vi "EOL All-Station Module Test Data Buffer.vi"() -> (1 "Store Data out":T1 {"Sun Shade Open Force Limits"."Variance" format="%.2g"; "Sun Shade Open Force Limits"."Truncation End" format="%.2g"; "Sun Shade Open Force Limits"."Truncation Start" format="%.2g"; "Sun Shade Open Force Limits"."Avg Max" format="%.2g"; "Sun Shade Open Force Limits"."Avg Min" format="%.2g"; "Sun Shade Open Force Limits"."Overall Max" format="%.2g"; "Sun Shade Open Force Limits"."Overall Min" format="%.2g"; "Sun Shade Close Force Limits"."Variance" format="%.2g"; "Sun Shade Close Force Limits"."Truncation End" format="%.2g"; "Sun Shade Close Force Limits"."Truncation Start" format="%.2g"; "Sun Shade Close Force Limits"."Avg Max" format="%.2g"; "Sun Shade Close Force Limits"."Avg Min" format="%.2g"; "Sun Shade Close Force Limits"."Overall Max" format="%.2g"; "Sun Shade Close Force Limits"."Overall Min" format="%.2g"; "Motion Data Array"."Motion Data Limits"."LIN Msg"."Msg" format="%02x"; "Motion Data Array"."Motion Data Limits"."LIN Msg"."ID" format="%02x"})   [LabVIEW 2018]
uses:
  02.Type Def's/EOL Save Module Test Data Control.ctl
  02.Type Def's/EOL Motion Database Table.ctl
  02.Type Def's/All Motions.ctl
  05.UserVI's/type defs/17x Audit Motion Data Seq Control.ctl
  05.UserVI's/type defs/17x AP Data Type.ctl
  05.UserVI's/type defs/17x Sunshade Limts Seq.ctl
  02.Type Def's/EOL Module Info Control.ctl
panel:
  # "Min"
  # "N"
  # "Min"
  # "Start"
  # "N"
  # "Max"
  # "N"
  # "Max"
  # "N"
  # "End"
  # "Min"
  # "N"
  # "Min"
  # "Start"
  # "N"
  # "Max"
  # "N"
  # "Max"
  # "N"
  # "End"
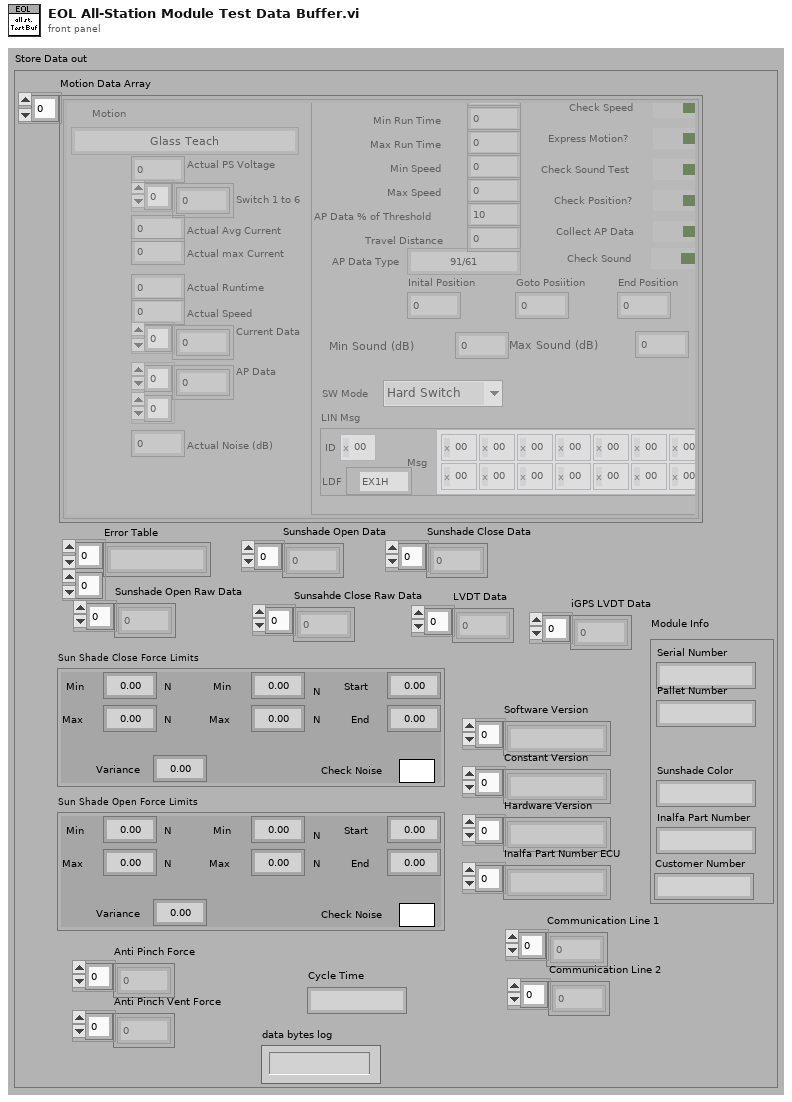
[diagram p1: front panel]
types:
  T1 = typedef "EOL Save Module Test Data Control.ctl" = cluster{"Motion Data Array":T2[], "Error Table":string[][], "Sun Shade Close Force Limits":T6, "Sun Shade Open Force Limits":T6, "Sunshade Open Data":sgl[], "Sunshade Close Data":sgl[], "Module Info":T7, "Sunsahde Close Raw Data":sgl[], "Sunshade Open Raw Data":sgl[], "Software Version":string[], "Constant Version":string[], "Hardware Version":string[], "Inalfa Part Number ECU":string[], "LVDT Data":sgl[], "Communication Line 1":sgl[], "Communication Line 2":sgl[], "Anti Pinch Force":sgl[], "Cycle Time":string, "Anti Pinch Vent Force":sgl[], "iGPS LVDT Data":sgl[], "data bytes log":string}
  T2 = typedef "EOL Motion Database Table.ctl" = cluster{"Motion":T3, "Actual Avg Current":dbl, "Actual Runtime":dbl, "Actual Speed":dbl, "Current Data":sgl[], "Motion Data Limits":T4, "Switch 1 to 6":dbl[], "Actual PS Voltage":dbl, "AP Data":i16[][], "Actual max Current":dbl, "Actual Noise (dB)":dbl}
  T3 = typedef "All Motions.ctl" = enum16{"Glass Teach", "Glass Slide Open", "Glass Slide Close", "Glass Vent Open", "Glass Vent Close", "Sunshade Teach", "Sunshade Open", "Sunshade Close", "Idle", "Sunshade Open 2", "Sunshade Close 2", "Glass Slide Open Sunshade Open", "Glass Slide Open Sunshade Close", "Glass Slide Close Sunshade Open", "Glass Slide Close Sunshade Close", "Glass Vent Open Sunshade Open", "Glass Vent Open Sunshade Close", "Glass Vent Close Sunshade Open", "Glass Vent Close Sunshade Close", "Express Glass Slide Open", "Express Glass Slide Close", "Express Glass Vent Open", "Express Glass Vent Close", "Express Sunshade Open", "Express Sunshade Close", "Express Sunshade Open 2", "Express Sunshade Close 2", "Express Glass Slide Open Sunshade Open", "Express Glass Slide Open Sunshade Close", "Express Glass Slide Close Sunshade Open", "Express Glass Slide Close Sunshade Close", "Express Glass Vent Open Sunshade Open", "Express Glass Vent Open Sunshade Close", "Express Glass Vent Close Sunshade Open", "Express Glass Vent Close Sunshade Close", "Goto Position Glass", "Goto Position Sunshade", "Sunshade Teach 2"}
  T4 = typedef "17x Audit Motion Data Seq Control.ctl" = cluster{"Power Supply Voltage":dbl, "Min Avg Current":dbl, "Max Avg Current":dbl, "Min Run Time":dbl, "Max Run Time":dbl, "Min Speed":dbl, "Max Speed":dbl, "AP Data % of Threshold":dbl, "Travel Distance":dbl, "AP Data Type":T5, "Check Current":bool, "Check Run Time":bool, "Check Speed":bool, "Express Motion?":bool, "Check Sound Test":bool, "Check Position?":bool, "Collect AP Data":bool, "Inital Position":u16, "End Position":u16, "Goto Posiition":u16, "Max max Current":dbl, "Min max Current":dbl, "Check max Current":bool, "Check Sound":bool, "Min Sound (dB)":dbl, "Max Sound (dB)":dbl, "SW Mode":enum16{"Hard Switch", "Uncond Frame"}, "LIN Msg":cluster{"ID":u8, "Msg":u8[][], "LDF":refnum<k21>}}
  T5 = typedef "17x AP Data Type.ctl" = enum16{"91/61", "92/62", "93/63", "67", "68", "6F", "71", "91 Msg", "92 Msg", "93 Msg", "94 Msg", "HiRain 91", "HiRain 92 Speed", "HiRain 92 HS", "HiRain 92", "HiRain 93", "SnT"}
  T6 = typedef "17x Sunshade Limts Seq.ctl" = cluster{"Overall Min":dbl, "Overall Max":dbl, "Avg Min":dbl, "Avg Max":dbl, "Truncation Start":dbl, "Truncation End":dbl, "Variance":dbl, "Check Noise":bool}
  T7 = typedef "EOL Module Info Control.ctl" = cluster{"Serial Number":string, "Pallet Number":string, "Sunshade Color":string, "Inalfa Part Number":string, "Customer Number":string}
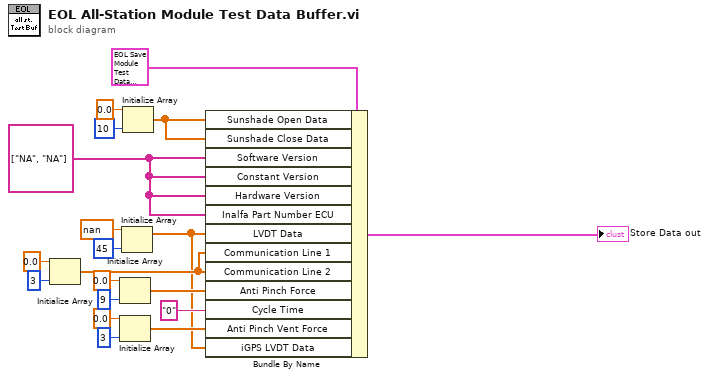
[diagram p0: block diagram]
diagram:
  w14 = string[] ["NA", "NA"] ("Software Version")
  n1 = Initialize Array(sgl 0.0 ("element"), 3 ("dimension size")) -> (w9:sgl[])
  n2 = Initialize Array(sgl 0.0 ("element"), 9 ("dimension size")) -> (w6:sgl[])
  n3 = Initialize Array(sgl 0.0 ("element"), 3 ("dimension size")) -> (w2:sgl[])
  n4 = Initialize Array(sgl nan ("element"), 45 ("dimension size")) -> (w1:sgl[])
  n5 = Initialize Array(sgl 0.0 ("element"), 10 ("dimension size")) -> (w15:sgl[])
  n6 = Bundle By Name(cluster=T1 {"Motion Data Array"=[], "Error Table"=[], "Sun Shade Close Force Limits"={"Overall Min"=0.0, "Overall Max"=0.0, "Avg Min"=0.0, "Avg Max"=0.0, "Truncation Start"=0.0, "Truncation End"=0.0, "Variance"=0.0, "Check Noise"=FALSE}, "Sun Shade Open Force Limits"={"Overall Min"=0.0, "Overall Max"=0.0, "Avg Min"=0.0, "Avg Max"=0.0, "Truncation Start"=0.0, "Truncation End"=0.0, "Variance"=0.0, "Check Noise"=FALSE}, "Sunshade Open Data"=[], "Sunshade Close Data"=[], "Module Info"={"Serial Number"="", "Pallet Number"="", "Sunshade Color"="", "Inalfa Part Number"="", "Customer Number"=""}, "Sunsahde Close Raw Data"=[], "Sunshade Open Raw Data"=[], "Software Version"=[], "Constant Version"=[], "Hardware Version"=[], "Inalfa Part Number ECU"=[], "LVDT Data"=[], "Communication Line 1"=[], "Communication Line 2"=[], "Anti Pinch Force"=[], "Cycle Time"="", "Anti Pinch Vent Force"=[], "iGPS LVDT Data"=[], "data bytes log"=""} ("Audit Store Data"), "Sunshade Open Data"=w15, "Sunshade Close Data"=w15, "Software Version"=w14, "Constant Version"=w14, "Hardware Version"=w14, "Inalfa Part Number ECU"=w14, "LVDT Data"=w1, "Communication Line 1"=w9, "Communication Line 2"=w9, "Anti Pinch Force"=w6, "Cycle Time"="0", "Anti Pinch Vent Force"=w2, "iGPS LVDT Data"=w1) -> (→"Store Data out":T1)
